vi "WPI_Gyro_ADXRS453_ReadSensorData_3005.vi"(8 "error in (no error)":errorcluster, 9 "Sequence":u8, 11 "SPIDevRef in":T1) -> (0 "error out":errorcluster, 1 "Sequence Out (n-1)":u8, 2 "Sensor Data (n-1)":i16, 3 "SPIDevRef out":T1, 4 "Data Good":bool)   [LabVIEW 2016, in "Path Track.lvlib"]
uses:
  Path Track.lvlib
  <vilib>/Rock Robotics/WPI/SPI/WPI_SPIDevRef.ctl
  <vilib>/Rock Robotics/SystemInterfaces/spilib/spi_bus.ctl
  <vilib>/Rock Robotics/WPI/Gyro/ADXRS453/WPI_Gyro_ADXRS453_Commands.ctl
  <vilib>/Rock Robotics/WPI/Gyro/ADXRS453/WPI_Gyro_ADXRS453_Status.ctl
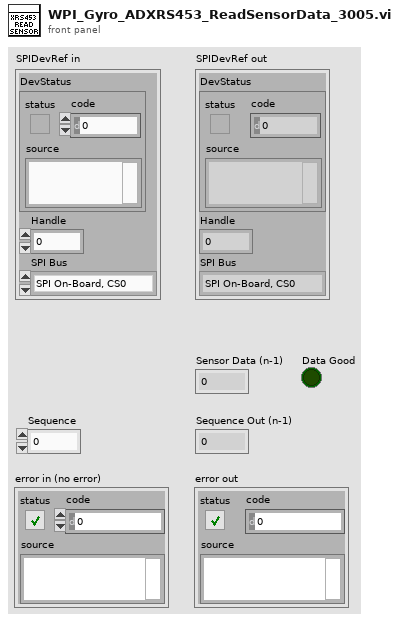
[diagram p1: front panel]
types:
  T1 = typedef "WPI_SPIDevRef.ctl" = cluster{"DevStatus":errorcluster, "Handle":i32, "SPI Bus":T2}
  T2 = typedef "spi_bus.ctl" = enum16{"SPI On-Board, CS0", "SPI On-Board, CS1", "SPI On-Board, CS2", "SPI On-Board, CS3", "SPI MXP", "Invalid"}
  T3 = typedef "WPI_Gyro_ADXRS453_Commands.ctl" = u8
  T4 = typedef "WPI_Gyro_ADXRS453_Status.ctl" = enum8{"Invalid", "Valid", "Self-Test", "Read/Write"}
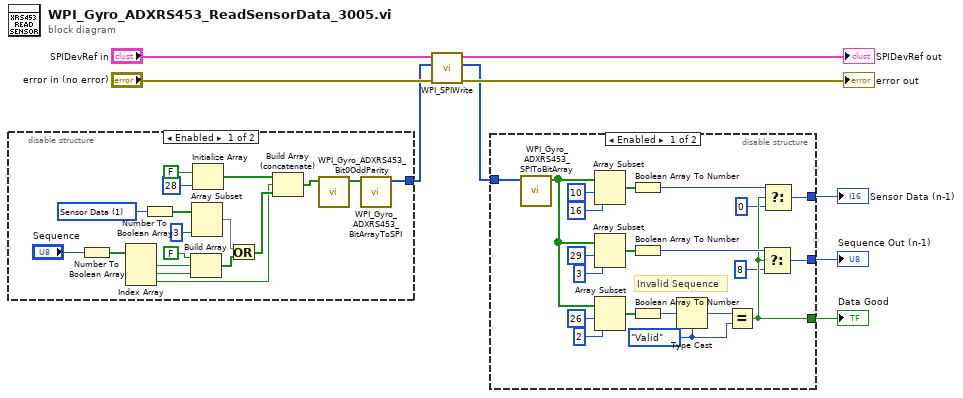
[diagram p0: block diagram]
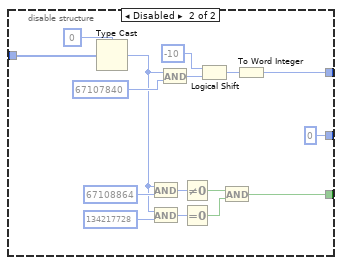
[diagram p2: hidden frame]
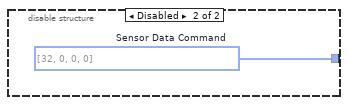
[diagram p3: hidden frame]
diagram:
  n1 = disable-structure shown="Enabled" {
    disable-tunnel: [w12 w28] -> w4
    frame Enabled {
      w20 = T3 1 items=["Read"=4, "Write"=2, "Sensor Data"=1]
      n2 = Number To Boolean Array(number="Sequence") -> (Boolean array=w18:bool[])
      n3 = Index Array(array=w18) -> (element #1=w17:bool, element #2=w16:bool, element #3=w10:bool)  [unwired: 3 in]
      n4 = Number To Boolean Array(number=w20) -> (Boolean array=w21:bool[])
      n5 = Build Array(FALSE, w17, w16) -> (w14:bool[])
      n6 = Array Subset(array=w21, length=3) -> (w13:bool[])  [unwired: 1 in]
      n7 = Initialize Array(FALSE, 28 ("dimension size")) -> (w26:bool[])
      n8 = Or(x=w13, y=w14) -> (x .or. y?=w11:bool[])
      n9 = Build Array (concatenate)(w26, w10, w11) -> (w25:bool[])
      n10 = call <vilib>:"WPI_Gyro_ADXRS453_Bit0OddParity.vi"("Array in"=w25) -> ("Array out"=w27:bool[])  [unwired: 10 in]
      n11 = call <vilib>:"WPI_Gyro_ADXRS453_BitArrayToSPI.vi"("32-bit Array in"=w27) -> ("SPI Byte Array (MSB first)"=w12:u8[])  [unwired: 10 in]
    }
    frame Disabled {
      w28 = u8[] [32, 0, 0, 0]  # Sensor Data Command
    }
  }
  n12 = call <vilib>:"WPI_SPIWrite.vi"("error in (no error)"="error in (no error)", "Data To Send"=w4, "SPIDevRef"="SPIDevRef in") -> ("error out"=→"error out":errorcluster, "Received Data"=w5:u8[], "SPIDevRef"=→"SPIDevRef out":T1)  [unwired: 6 out]
  n13 = disable-structure shown="Enabled" {
    disable-tunnel: w5 -> [w43 w62]
    disable-tunnel: [w35 u8 0 ("Sequence Out (n-1)")] -> w3
    disable-tunnel: [w34 w51] -> w2
    disable-tunnel: [w31 w56] -> w1
    frame Enabled {
      w36 = WPI_Gyro_ADXRS453_Status."Valid"
      # "Invalid Sequence"
      n14 = call <vilib>:"WPI_Gyro_ADXRS453_SPIToBitArray.vi"("SPI Byte Array (MSB first)"=w43) -> ("32-bit Boolean array"=w40:bool[])  [unwired: 10 in]
      n15 = Array Subset(array=w40, index=10, length=16) -> (w49:bool[])
      n16 = Array Subset(array=w40, index=29, length=3) -> (w44:bool[])
      n17 = Array Subset(array=w40, index=26, length=2) -> (w39:bool[])
      n18 = Boolean Array To Number(Boolean array=w49) -> (number=w33:i16)
      n19 = Boolean Array To Number(Boolean array=w44) -> (number=w32:u8)
      n20 = Boolean Array To Number(Boolean array=w39) -> (number=w38:u8)
      n21 = Type Cast(type=w36, x=w38) -> (*(type *) &x=w37:T4)
      n22 = Equal?(x=w37, y=w36) -> (x = y?=w31:bool)
      n23 = Select(t=w32, s=w31, f=u8 8) -> (s? t:f=w35:u8)
      n24 = Select(t=w33, s=w31, f=i16 0) -> (s? t:f=w34:i16)
    }
    frame Disabled {
      n25 = Type Cast(type=u32 0 ("y"), x=w62) -> (*(type *) &x=w50:u32)
      n26 = And(x=w50, y=u32 67108864) -> (x .and. y?=w63:u32)
      n27 = And(x=w50, y=u32 134217728) -> (x .and. y?=w59:u32)
      n28 = And(x=w50, y=u32 67107840) -> (x .and. y?=w54:u32)
      n29 = Not Equal To 0?(x=w63) -> (x != 0?=w60:bool)
      n30 = Equal To 0?(x=w59) -> (x = 0?=w57:bool)
      n31 = Logical Shift(y=i16 -10, x=w54) -> (x << y=w52:u32)
      n32 = And(x=w60, y=w57) -> (x .and. y?=w56:bool)
      n33 = To Word Integer(number=w52) -> (16bit integer=w51:i16)
    }
  }
  "Data Good" <- w1
  "Sensor Data (n-1)" <- w2
  "Sequence Out (n-1)" <- w3
